vi "Done FreeType.vi"(8 "error in (no error)":errorcluster, 11 "library in":i64) -> (0 "error out":errorcluster)   [LabVIEW 2023, in "Freetype Drawer.lvlib"]
uses:
  Freetype Drawer.lvlib
  libfreetype.dll
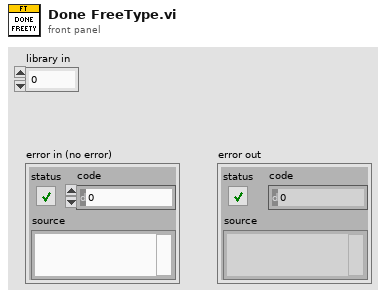
[diagram p1: front panel]
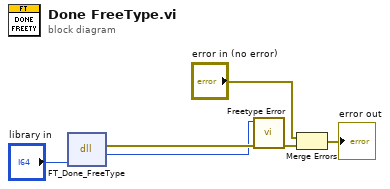
[diagram p0: block diagram]
diagram:
  n1 = dll-call lib="E:/Labview/LV 2023/Libs/LV Symbol/Freetype Drawer/Wrappers/libfreetype.dll" fn="FT_Done_FreeType"("library"="library in") -> (error out=w2:errorcluster, "error"=w1:i32)  [unwired: 4 in, 1 out]
  n2 = call "Freetype Error.vi"("error in (no error)"=w2, "Error"=w1) -> ("error out"=w3:errorcluster)  [unwired: 9 in]
  n3 = Merge Errors("error in (no error)", w3) -> (→"error out":errorcluster)
